vi "Configure Ramping.vi"(7 "Duration (1 min)":dbl=1.0 min=0.0, 8 "error in (no error)":errorcluster, 9 "End rate (1 ml/min)":dbl=1.0, 10 "Start rate (0 ml/min)":dbl, 11 "VISA resource name":refnum<visa-resource-name>) -> (0 "error out":errorcluster, 3 "VISA resource name out":refnum<visa-resource-name>)   [LabVIEW 2018]
panel:
  out "resulting string":string
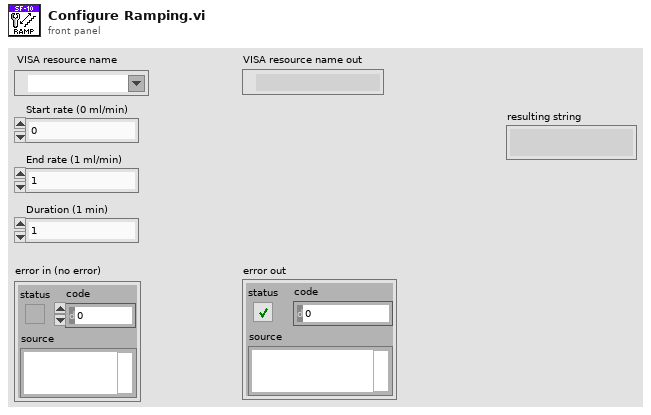
[diagram p1: front panel]
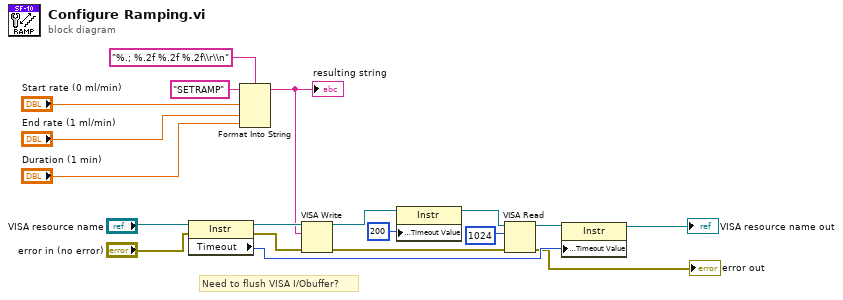
[diagram p0: block diagram]
diagram:
  # "Need to flush VISA I/Obuffer?"
  n1 = property class="Instr"(reference="VISA resource name", error in="error in (no error)") -> (reference out=w12:refnum<visa-resource-name>, error out=w10:errorcluster, "Timeout"=w2:u32)
  n2 = Format Into String(format string="%.; %.2f %.2f %.2f\\r\\n", initial string="SETRAMP", "Start rate (0 ml/min)", "End rate (1 ml/min)", "Duration (1 min)") -> (resulting string=w11:string)  [unwired: 1 in, 1 out]
  "resulting string" <- w11
  n3 = VISA Write(VISA resource name=w12, write buffer=w11, error in (no error)=w10) -> (VISA resource name out=w6:refnum<visa-resource-name>, error out=w5:errorcluster)  [unwired: 1 out]
  n4 = property class="Instr"(reference=w6, "General Settings:Timeout Value"=u32 200) -> (reference out=w9:refnum<visa-resource-name>)  [unwired: 1 in, 1 out]
  n5 = VISA Read(VISA resource name=w9, byte count=u32 1024, error in (no error)=w5) -> (VISA resource name out=w3:refnum<visa-resource-name>, error out=→"error out":errorcluster)  [unwired: 2 out]
  n6 = property class="Instr"(reference=w3, "General Settings:Timeout Value"=w2) -> (reference out=→"VISA resource name out":refnum<visa-resource-name>)  [unwired: 1 in, 1 out]
